vi "parse_chart_data.vi"(8 "error constant":errorcluster, 10 "swabian_data_in":i32[][](array[numeric]), 11 "active_channels":i32[](array[numeric])) -> (0 "error constant 2":errorcluster, 2 "formatted_data":i32[](array[numeric]), 3 "active_channels_out":i32[](array[numeric]))   [LabVIEW 2018]
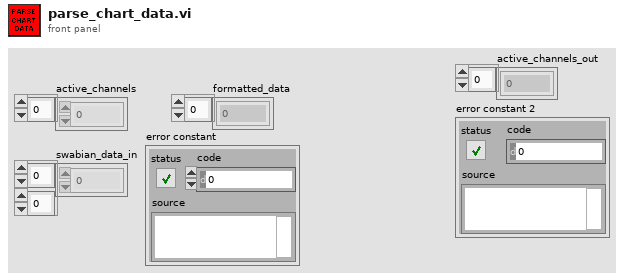
[diagram p1: front panel]
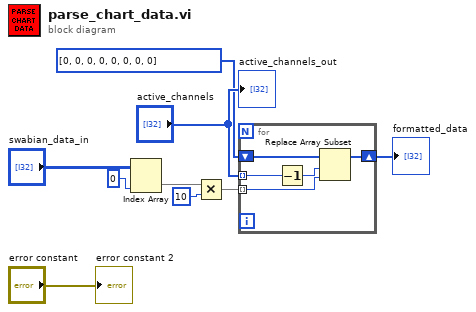
[diagram p0: block diagram]
diagram:
  n1 = Index Array(array="swabian_data_in", index (col)=0 ("index (row)")) -> (element=w3:i32[])  [unwired: 1 in]
  n2 = Multiply(x=w3, y=10) -> (x*y=w7:i32[])
  n3 = for {
    shift-right: [w13] -> w9
    shift-left: i32[] [0, 0, 0, 0, 0, 0, 0, 0] ("Array in") -> [w14]
    tunnel: w7 -> [w12] mode=indexing
    tunnel: "active_channels" -> [w11] mode=indexing
    n4 = Decrement(x=w11) -> (x-1=w10:i32)
    n5 = Replace Array Subset(array=w14, new element=w12, index=w10) -> (w13:i32[])
  }
  "formatted_data" <- w9
  "active_channels_out" <- "active_channels"
  "error constant 2" <- "error constant"
